vi "camera_acquisition_sequence.vi"(0 "Session In":T2 caption="Camera In", 1 "Desired image number":i32=1, 2 "error in":errorcluster) -> (3 "Session Out":T2 caption="Camera Out", 4 "Image Array":T1[](array[typedef]), 6 "error out":errorcluster)   [LabVIEW 2009]
uses:
  <vilib>/userDefined/High Color/IMAQdx.ctl
  <vilib>/vision/Image Controls.llb/IMAQ Image.ctl
  <vilib>/vision/driver/IMAQdx.llb/IMAQdx Acquisition Mode.ctl
  <vilib>/vision/driver/IMAQdx.llb/IMAQdx Buffer Number Mode.ctl
  <vilib>/vision/driver/NI_Vision_Acquisition_Software.lvlib
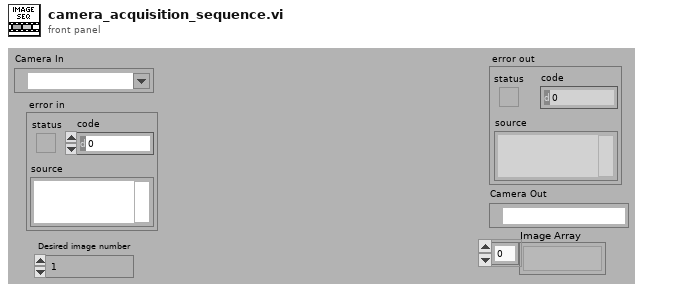
[diagram p1: front panel]
types:
  T1 = typedef "IMAQ Image.ctl" = refnum<image>
  T2 = typedef "IMAQdx.ctl" = refnum<k21>
  T3 = typedef "NI_Vision_Acquisition_Software.lvlib/IMAQdx Acquisition Mode.ctl" = enum32{"One Shot", "Continuous"}
  T4 = typedef "Image Type" = u32
  T5 = typedef "NI_Vision_Acquisition_Software.lvlib/IMAQdx Buffer Number Mode.ctl" = enum32{"Next", "Last", "Buffer Number"}
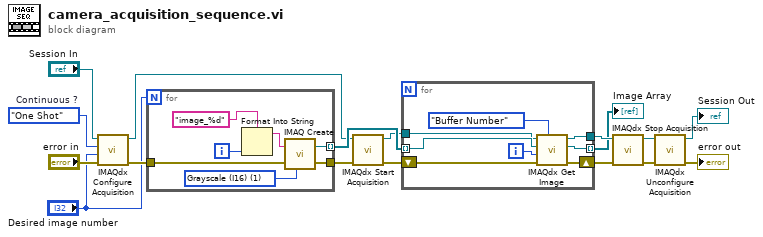
[diagram p0: block diagram]
diagram:
  w7 = IMAQdx_Acquisition_Mode."One Shot"  # Continuous ?
  n1 = call <vilib>:"IMAQdx Configure Acquisition.vi"("error in"="error in", "Number of Buffers"="Desired image number", "Continuous?"=w7, "Session In"="Session In") -> ("error out"=w8:errorcluster, "Session Out"=w9:T2)  [unwired: 6 out]
  n2 = for {
    N: "Desired image number" -> [_]
    tunnel: w8 -> [w24]
    tunnel: [w23] -> w12 mode=indexing
    tunnel: [w22] -> w10
    i -> [w21]
    w18 = T4 1 items=["Grayscale (U8)", "Grayscale (I16)", "Grayscale (SGL)", "Complex (CSG)", "RGB (U32)", "HSL (U32)", "RGB (U64)", "Grayscale (U16)"] ("Image Type")
    n3 = Format Into String(format string="image_%d" ("Image Name"), w21) -> (resulting string=w20:string)  [unwired: 2 in, 1 out]
    n4 = call "IMAQ Create"("Image Name"=w20, "Image Type"=w18, "error in (no error)"=w24) -> ("New Image"=w23:T1, "error out"=w22:errorcluster)  [unwired: 1 in, 1 out]
  }
  n5 = call <vilib>:"IMAQdx Start Acquisition.vi"("error in"=w10, "Session In"=w9) -> ("error out"=w13:errorcluster, "Session Out"=w11:T2)  [unwired: 8 out]
  n6 = for {
    tunnel: w12 -> [w32] mode=indexing
    shift-right: [w30] -> w14
    shift-left: w13 -> [w31]
    tunnel: [w29] -> w15
    tunnel: w11 -> [w28]
    tunnel: [w27] -> w1 mode=indexing
    i -> [w25]
    n7 = call <vilib>:"IMAQdx Get Image.vi"("Buffer Number Mode (Next)"=IMAQdx_Buffer_Number_Mode."Buffer Number", "error in"=w31, "Buffer Number In"=w25, "Image In"=w32, "Session In"=w28) -> ("error out"=w30:errorcluster, "Image Out"=w27:T1, "Session Out"=w29:T2)  [unwired: 4 out]
  }
  "Image Array" <- w1
  n8 = call <vilib>:"IMAQdx Stop Acquisition.vi"("error in"=w14, "Session In"=w15) -> ("error out"=w16:errorcluster, "Session Out"=w17:T2)  [unwired: 8 out]
  n9 = call <vilib>:"IMAQdx Unconfigure Acquisition.vi"("error in"=w16, "Session In"=w17) -> ("error out"=→"error out":errorcluster, "Session Out"=→"Session Out":T2)  [unwired: 8 out]
